vi "Timed Loop and Occurrence.vi"() -> ()   [LabVIEW 2012]
uses:
  <vilib>/Platform/TimedLoop/XDataNode/timing_clust.ctl
  <vilib>/Platform/TimedLoop/XDataNode/nitl_modes.ctl
  <vilib>/Platform/TimedLoop/XDataNode/wakeup.ctl
  <vilib>/platform/TimedLoop/XDataNode/XDataNode.xnode
  <vilib>/Platform/TimedLoop/XDataNode/XDNodeRunTimeDep.lvlib
panel:
  in  "Generate Occurence?":bool
  out "Occurence":i32
  out "Timed Loop":i32
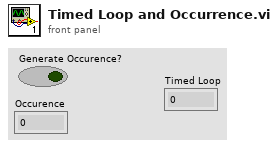
[diagram p1: front panel]
types:
  T1 = typedef "XDNodeRunTimeDep.lvlib/timing_clust.ctl" = cluster{"Expected End [f-1]":u64, "Actual End [f-1]":u64, "Finished Late? [f-1]":bool, "Expected End [i-1]":u64, "Actual End [i-1]":u64, "Finished Late? [i-1]":bool, "Expected Start [i]":u64, "Actual Start [i]":u64, "Expected Start [f]":u64, "Actual Start [f]":u64, "Source Name":string, "Structure Name":string, "Period":i64, "Deadline":i64, "Offset":i64, "Start":i64, "Priority":i32, "Timeout":i32, "Mode":T2, "Wakeup Reason":T3, "Error":errorcluster, "Source Type":string, "Secondary Source Type":string, "Global End Time":u64, "Global Start Time":u64, "Frame Duration":u64, "Iteration Duration":u64, "Assigned CPU":i32, "I/O Scan Engine Mode":u32}
  T2 = typedef "XDNodeRunTimeDep.lvlib/nitl_modes.ctl" = enum32{"No Change", "Process missed periods, maintain original phase", "Discard missed periods, maintain original phase", "Process missed periods, ignore original phase", "Discard missed periods, ignore original phase"}
  T3 = typedef "XDNodeRunTimeDep.lvlib/wakeup.ctl" = enum32{"Normal", "Aborted", "Asynchronous wakeup", "Timing source error", "Timed loop error", "Timeout"}
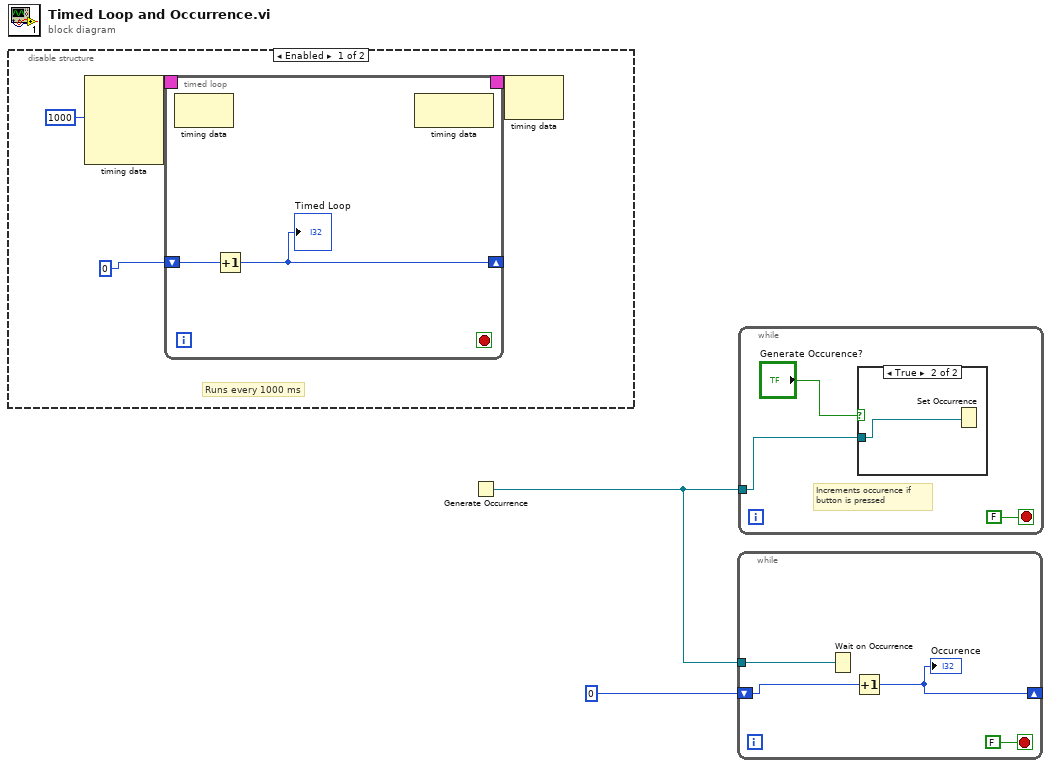
[diagram p0: block diagram]
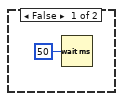
[diagram p2: hidden frame]
diagram:
  n1 = disable-structure shown="Enabled" {
    frame Enabled {
      # "Runs every 1000 ms"
      n2 = node-c288(i64 1000 ("Period")) -> (w6:T1)  [unwired: 3 in]
      n3 = timed-loop {
        timing: w6 -> [_]
        timing-out: [_] -> w5
        shift-right: [w7] -> _
        shift-left: 0 -> [w8]
        stop <- _ stop-if-true
        n4 = node-c288() -> ()  [unwired: 1 in, 1 out]
        n5 = Increment(x=w8) -> (x+1=w7:i32)
        "Timed Loop" <- w7
        n6 = node-c288() -> ()  [unwired: 1 in, 1 out]
      }
      n7 = node-c288(w5) -> ()  [unwired: 1 out]
    }
    frame Disabled {
    }
  }
  n8 = Generate Occurrence() -> (w1:refnum<k4>)
  n9 = while {
    shift-right: [w16] -> _
    shift-left: 0 -> [w17]
    tunnel: w1 -> [w15]
    stop <- FALSE stop-if-true
    n10 = Wait on Occurrence(2:w15) -> ()  [unwired: 2 in, 1 out]
    n11 = Increment(x=w17) -> (x+1=w16:i32)
    "Occurence" <- w16
  }
  n12 = while {
    tunnel: w1 -> [w20]
    stop <- FALSE stop-if-true
    # "Increments occurence if\nbutton is pressed"
    n13 = case shown="True" "Generate Occurence?" {
      tunnel: w20 -> [_ w23]
      frame False {
        n14 = Wait (ms)(milliseconds to wait=u32 50) -> ()  [unwired: 1 out]
      }
      frame True {
        n15 = Set Occurrence(w23) -> ()
      }
    }
  }
